vi "Set UDP and wait TCP value in range.vi"(6 "timeout":u32=30000, 8 "error in (no error)":errorcluster, 9 "tolerance":dbl=0.1 format="%#_13g", 10 "set value":dbl format="%#_13g", 11 "device and variable":string[](array[string])=["IP2-TC-ESP3", "Position.Axis 3"]) -> (0 "error out":errorcluster, 3 "In range is True":bool)   [LabVIEW 2020]
panel:
  out "x > y?":bool
  out "millisecond timer value":u32
  out "In Range?":bool
  out "No errors =T":bool
  out "Array":dbl[](array[numeric])
  out "Gossip out time":u32
  out "Gossip position":dbl
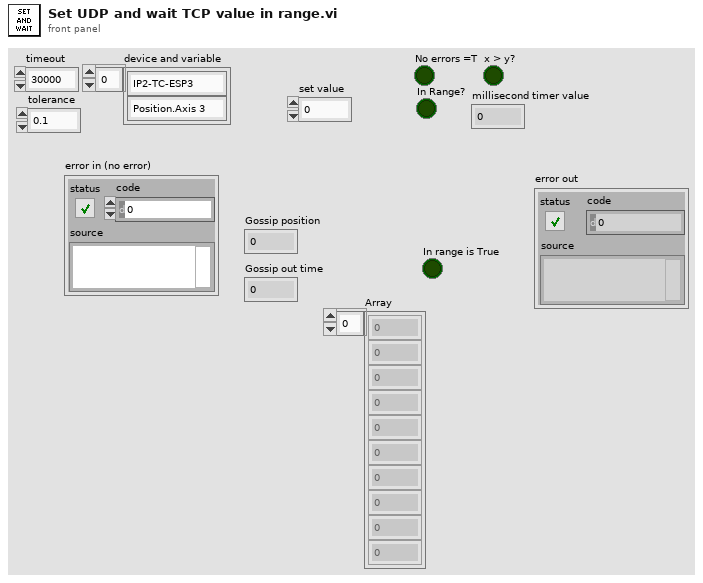
[diagram p1: front panel]
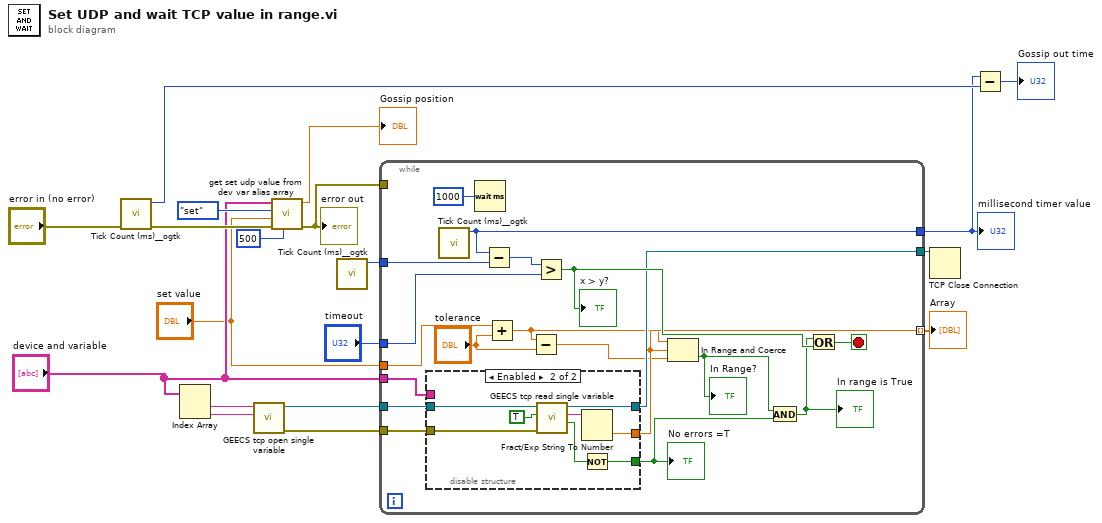
[diagram p0: block diagram]
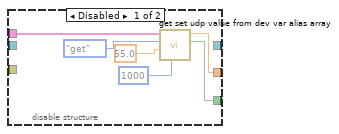
[diagram p2: hidden frame]
diagram:
  n1 = call <userlib>:"Tick Count (ms)__ogtk.vi"("error in (no error)"="error in (no error)") -> ("error out"=w13:errorcluster, "millisecond timer value"=w16:u32)  [unwired: 9 in]
  n2 = Index Array(array="device and variable") -> (element #1=w6:string, element #2=w5:string)  [unwired: 2 in]
  n3 = call "GEECS tcp open single variable.vi"("Variable name"=w5, "Device name"=w6) -> ("error out"=w4:errorcluster, "TCP Network Connection out"=w8:refnum<k5>)  [unwired: 7 in, 1 out]
  n4 = call "get set udp value from dev var alias array.vi"("slow timeout ms (3000)"=500, "error in (no error)"=w13, "Set position"="set value", "get or set"=enum16{"get", "set"}."set", "device and variable"="device and variable") -> ("error out"=w11:errorcluster, "Numeric"=→"Gossip position":dbl)  [unwired: 4 in, 1 out]
  "error out" <- w11
  n5 = call <userlib>:"Tick Count (ms)__ogtk.vi"() -> ("millisecond timer value"=w12:u32)  [unwired: 10 in, 1 out]
  n6 = while {
    tunnel: "device and variable" -> [w38]
    tunnel: w12 -> [w28]
    tunnel: w11 -> [_]
    tunnel: [w29] -> w10
    tunnel: [w33] -> w9 mode=indexing
    tunnel: w8 -> [w27]
    tunnel: w4 -> [w26]
    tunnel: [w25] -> w3
    tunnel: "timeout" -> [w24]
    tunnel: "set value" -> [w23]
    stop <- w36 stop-if-true
    n7 = disable-structure shown="Enabled" {
      disable-tunnel: w38 -> [w44 _]
      disable-tunnel: [w41 w48] -> w33
      disable-tunnel: [w39 w46] -> w31
      disable-tunnel: w27 -> [_ w51]
      disable-tunnel: w26 -> [_ w50]
      disable-tunnel: [_ w47] -> w25
      frame Disabled {
        n8 = call "get set udp value from dev var alias array.vi"("slow timeout ms (3000)"=1000, "Set position"=55.0, "get or set"=enum16{"get", "set"}."get", "device and variable"=w44) -> ("No errors =T"=w39:bool, "Numeric"=w41:dbl)  [unwired: 5 in, 1 out]
      }
      frame Enabled {
        n9 = call "GEECS tcp read single variable.vi"("error in (no error)"=w50, "clear buffer after read"=TRUE, "TCP Network Connection in"=w51) -> ("timed out"=w45:bool, "variable value"=w49:string, "TCP Network Connection out"=w47:refnum<k5>)  [unwired: 5 in, 1 out]
        n10 = Fract/Exp String To Number(string=w49) -> (number=w48:dbl)  [unwired: 3 in, 1 out]
        n11 = Not(x=w45) -> (.not. x?=w46:bool)
      }
    }
    "No errors =T" <- w31
    n12 = call <userlib>:"Tick Count (ms)__ogtk.vi"() -> ("millisecond timer value"=w29:u32)  [unwired: 10 in, 1 out]
    n13 = Wait (ms)(milliseconds to wait=u32 1000) -> ()  [unwired: 1 out]
    n14 = Subtract(x=w29, y=w28) -> (x-y=w37:u32)
    n15 = Add(x=w23, y="tolerance") -> (x+y=w22:dbl)
    n16 = Subtract(x=w22, y="tolerance") -> (x-y=w20:dbl)
    n17 = Greater?(x=w37, y=w24) -> (0:w35:bool)
    "x > y?" <- w35
    n18 = In Range and Coerce(upper limit=w22, x=w33, lower limit=w20) -> (In Range?=w32:bool)  [unwired: 1 out]
    "In Range?" <- w32
    n19 = And(x=w32, y=w31) -> (x .and. y?=w30:bool)
    "In range is True" <- w30
    n20 = Or(x=w30, y=w35) -> (x .or. y?=w36:bool)
  }
  "Array" <- w9
  "millisecond timer value" <- w10
  n21 = TCP Close Connection(connection ID=w3) -> ()  [unwired: 2 in, 2 out]
  n22 = Subtract(x=w10, y=w16) -> (x-y=→"Gossip out time":u32)
